vi "GlobalVariables.vi"() -> ()   [LabVIEW 2020]
panel:
  out "RightNoF":dbl
  out "LeftNoF":dbl
  out "flagNavxReset":bool
  out "StopShoot":bool
  out "Shoot":bool
  in  "Y":dbl[](array[numeric])
  in  "X":dbl[](array[numeric])
  out "PreviousY":dbl
  out "Mean":dbl
  out "Right":dbl
  out "Left":dbl
  out "YActual":dbl
  out "XActual":dbl
  out "AimingAdjust":dbl
  out "flagEncodersResets":bool
  out "Limeduslight":bool
  out "PreviousX":dbl
  out "ValidTarget":bool
  in  "Ty":dbl(slide) scale=-25.0..25.0
  out "Tx":dbl(knob) scale=-25.0..25.0
  out "MINslider":bool
  out "MAXslider":bool
  out "EncoderSlider":dbl
  out "Stop":bool
  out "Ultrassonic02_mm":u8(slide) scale=0.0..498.0
  out "Ultrassonic01_mm":u8(slide) scale=0.0..498.0
  out "Yaw":dbl(knob) scale=0.18..180.0
  out "Ultrassonic02_Inch":dbl
  out "Ultrassonic01_Inch":dbl
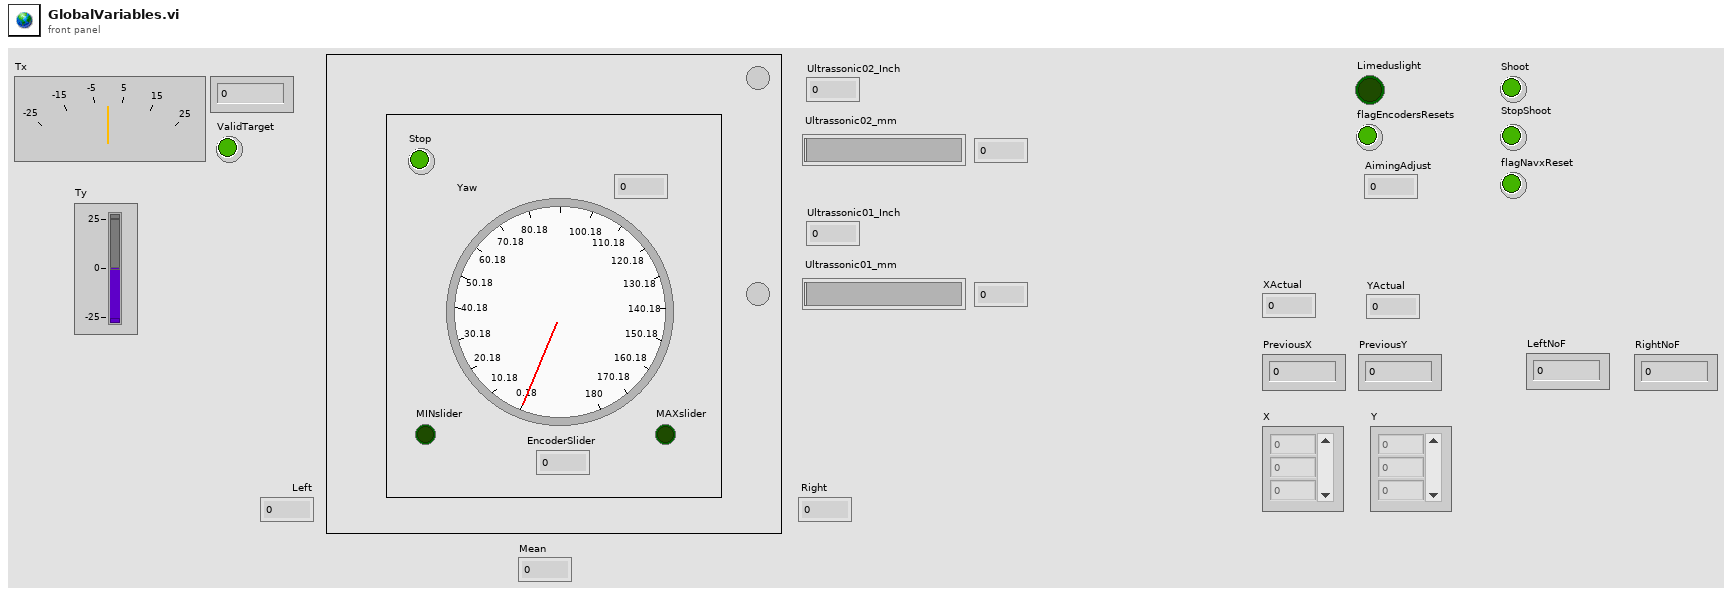
[diagram p1: front panel]
diagram:
